vi "Service.vi"() -> ()   [LabVIEW 2019, in "Service.lvlib"]
uses:
  Service.lvlib
  mmw_command_lib/src_LabVIEW/mmW_commands/TypeDefs/commands.ctl
  TypeDef/AppStates.ctl
  mmw_instr_app_api/instr app state.ctl
  <vilib>/Field R&D Services/Logger/Type Definitions/Severity.ctl
  MsgQ/TypeDefs/CommandsQ.ctl
  MsgQ/TypeDefs/MsgQ_Commands.ctl
  mmw_command_lib/src_LabVIEW/mmW_commands/TypeDefs/response status.ctl
  <vilib>/Field R&D Services/Logger/Support/Create Level String.vi
  <vilib>/Field R&D Services/Logger/Support/Strip Whitespace.vi
  <vilib>/dlg_ctls.llb/Space Constant.vi
  <vilib>/Utility/error.llb/Trim Whitespace.vi
  <vilib>/Field R&D Services/Logger/Support/Manager.vi
  mmw_command_lib/src_LabVIEW/mmW_commands/commands/extract_messages/extract_configure_fs.vi
  mmw_command_lib/src_LabVIEW/mmW_commands/commands/extract_messages/extract_get_instrument_status.vi
  mmw_command_lib/src_LabVIEW/mmW_commands/commands/construct_messages/construct_get_instrument_status.vi
  <vilib>/Field R&D Services/Logger/Support/Control State.vi
  MsgQ/MsgQ.lvlib
  <vilib>/Field R&D Services/Logger/Field_RnD_Services_Logger_Toolkit.lvlib
  mmw_command_lib/src_LabVIEW/mmW_commands/mmW_commands.lvlib
  zmq_multipart_lib/src_LabVIEW/zmq_mulipart_lib/zmq_multipart_lib.lvclass
  mmw_instr_app_api/mmW_instr_app_API.lvlib
panel:
  in  "send":bool
  out "Array":T1[](array[typedef])
  in  "stop?":bool
  in  "Tab Control":enum32{"Server setup", "Debug", "Test Commands"}(tab)=enum."Debug"
  out "error out":errorcluster
  out "Main INI path":string="C:\\ProgramData\\Noffz\\mmW_Service\\mmw_Service.ini"
  out "Messages":i32(listbox)
  in  "Send Command":bool
  in  "commands":T2=enum."configure_rf"
  out "fc (Hz)":dbl
  out "parts":string[](array[string])
  out "state":T3
  out "watchdog timer":timestamp
  # "NI mmWave Service Application"
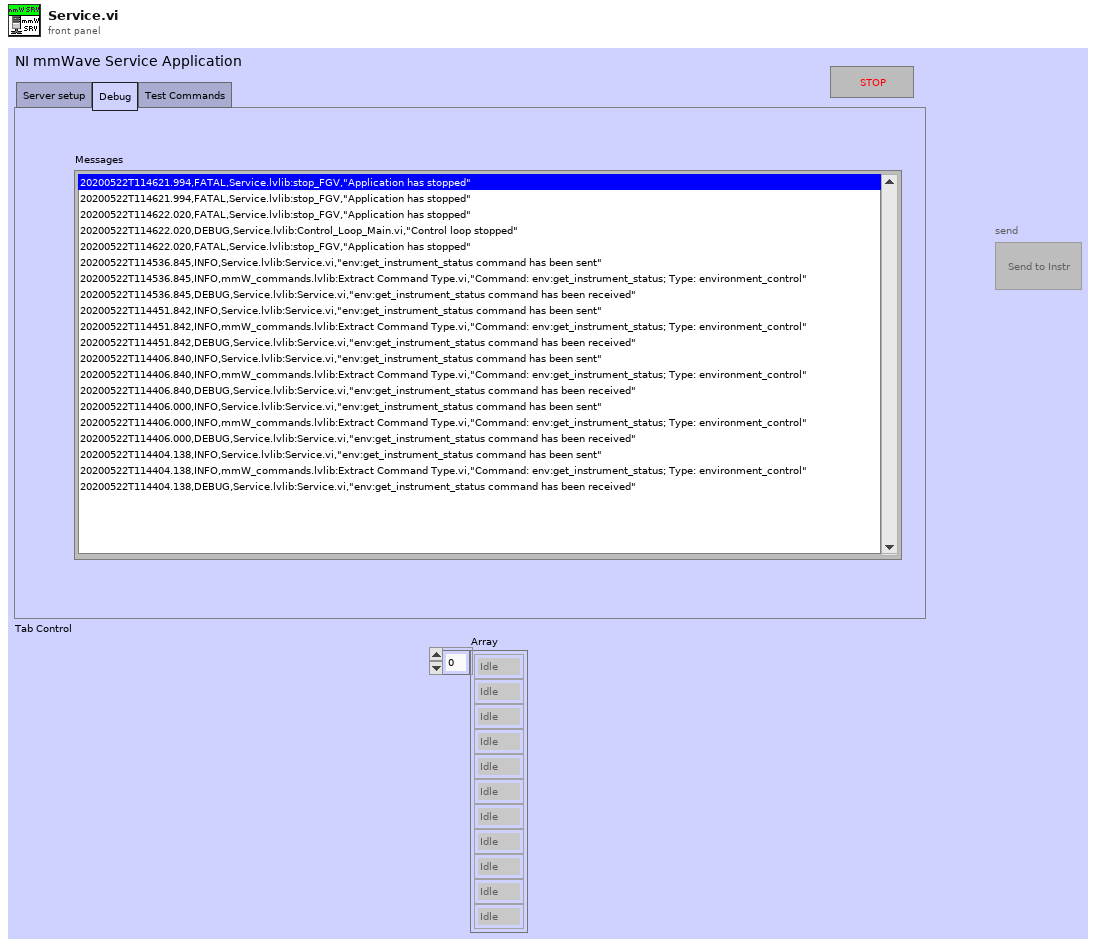
[diagram p1: front panel]
types:
  T1 = typedef "Service.lvlib/AppStates.ctl" = enum16{"Idle", "Init", "Proc_ZMQ_command", "Send_manual_command", "Shutdown", "Stop"}
  T2 = typedef "mmW_commands.lvlib/commands.ctl" = enum16{"configure_fs", "configure_rf", "configure_trigger", "equalization_enable", "equalization_start", "lo_sync_enable", "equalization_stop", "get_instrument_status", "get_versions", "initialize_hw", "pop_rx", "set_log_level", "Shutdown", "start", "start_instrument_app", "stop", "trans", "transceive", "trigger_burst", "trigger_sync_enable", "Write TX", "resp_generic", "resp_waveform", "send_trigger", "fetch", "transceive2"}
  T3 = typedef "mmW_instr_app_API.lvlib/instr app state.ctl" = enum16{"Off", "Initialization", "Configuration", "Running", "Calibration"}
  T4 = typedef "Field_RnD_Services_Logger_Toolkit.lvlib/Severity.ctl" = enum16{"Benign", "Warning", "Recoverable", "Fatal"}
  T5 = typedef "Service.lvlib/AppData.ctl" = cluster{"MsgQ":refnum<queue>, "Stop?":bool, "zmq sessions":cluster{"Control_endpoint":string, "Instr_endpoint":string}, "control-loop":cluster{"fromUI-Q":refnum<queue>, "toUI":refnum<user-event>, "Control_endpoint":string}, "UI-loop":cluster{"evnt_ref":refnum<event-registration>}, "logging":cluster{"level":dbl, "verbosity":dbl, "path":string, "Listener_ID":string}, "general_settings":cluster{"mmW_instr_ini_path":string, "mmW_instr_pid_path":string}}
  T6 = typedef "mmW_commands.lvlib/response status.ctl" = enum16{"OK", "Error", "Warning", "Unknown"}
  T7 = typedef "Service.lvlib/CommandsQ.ctl" = cluster{"cmd":T8, "data":variant, "notif":string}
  T8 = typedef "MsgQ.lvlib/MsgQ_Commands.ctl" = enum16{"message1", "message2", "message3", "generic", "transparent", "exception", "stop"}
  T9 = typedef "mmW_commands.lvlib/command_types.ctl" = enum16{"invalid_command", "instrument_control", "environment_control", "response"}
  T10 = typedef "Logger.lvlib/Statement.ctl" = cluster{"Time Stamp":timestamp, "Tag":T11, "Source":string, "Message":string}
  T11 = typedef "Logger.lvlib/Tag.ctl" = enum16{"Fatal", "Error", "Warn", "Info", "Debug", "Trace"}
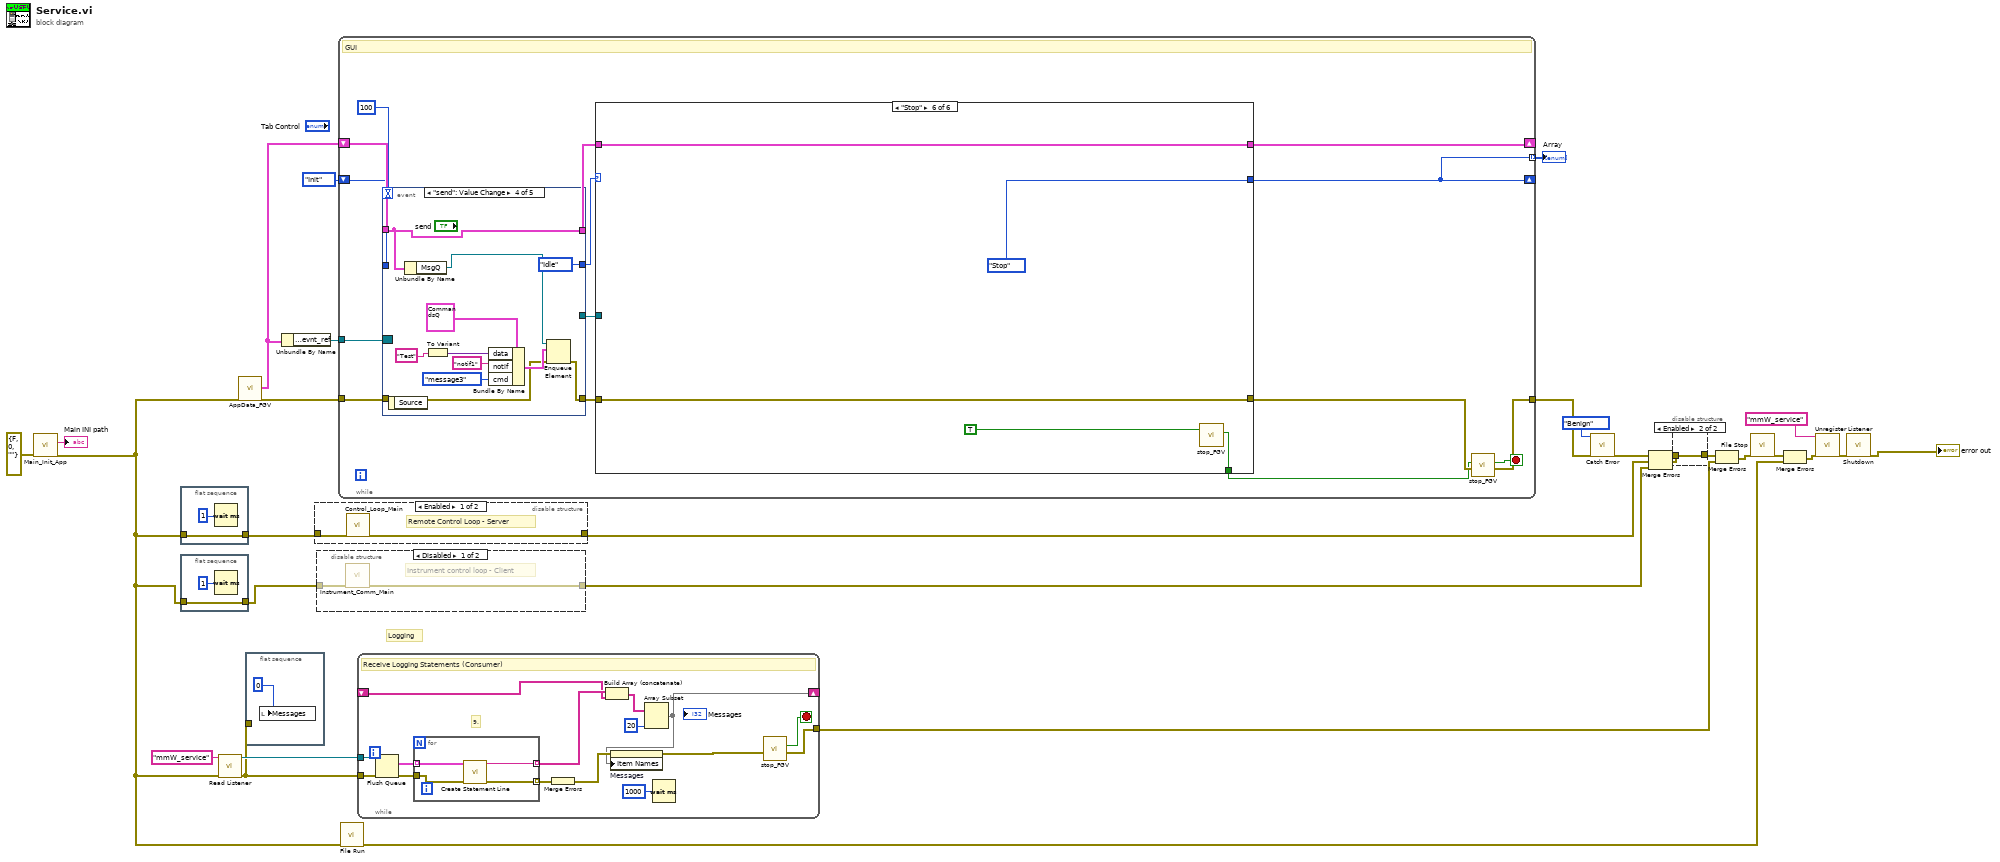
[diagram p0: block diagram]
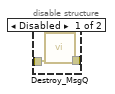
[diagram p3: hidden frame]
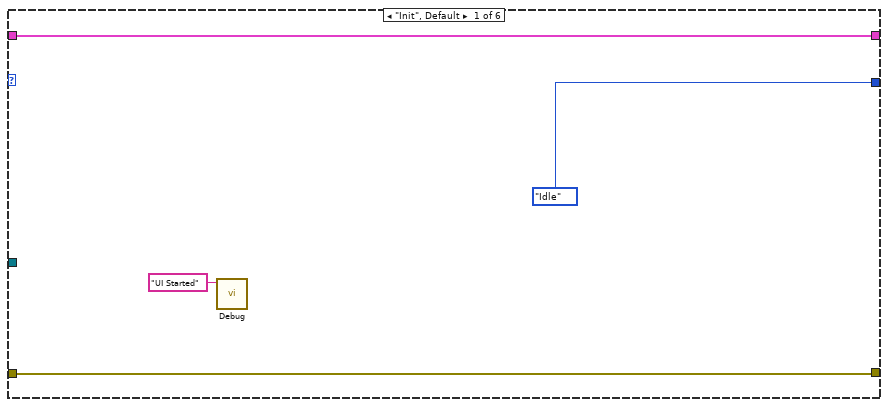
[diagram p5: hidden frame]
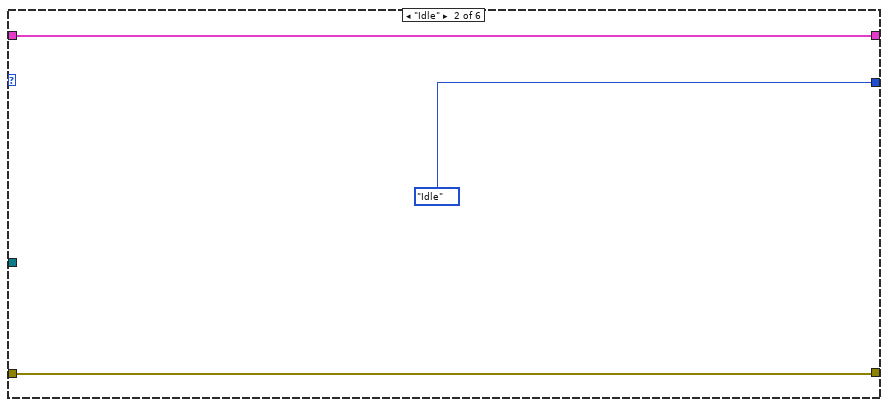
[diagram p6: hidden frame]
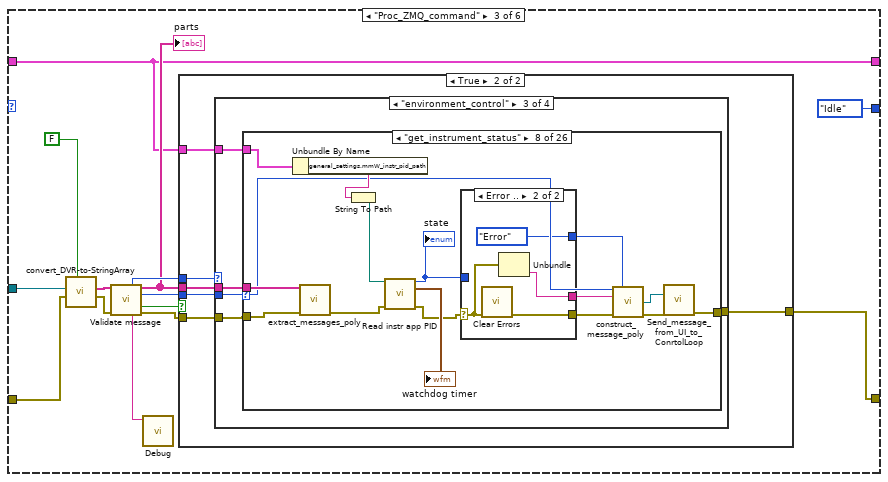
[diagram p7: hidden frame]
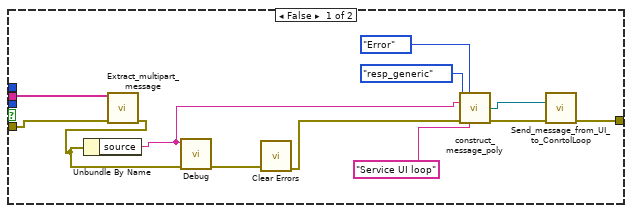
[diagram p8: hidden frame]
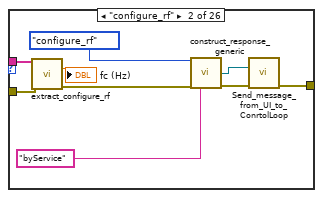
[diagram p12: hidden frame]
diagram:
  # "Logging"
  n1 = call "Main_Init_App.vi"("error in (no error)"=errorcluster {"status"=FALSE, "code"=0, "source"=""} ("Error In")) -> ("error out"=w3:errorcluster, "Main ini path"=→"Main INI path":string)  [unwired: 9 in]
  n2 = flat-sequence {
    tunnel: w3 -> [w30]
    tunnel: [w30] -> w4
    frame #0 {
      n3 = Wait (ms)(milliseconds to wait=u32 1) -> ()  [unwired: 1 out]
    }
  }
  n4 = flat-sequence {
    tunnel: w3 -> [w32]
    tunnel: [w32] -> w2
    frame #0 {
      n5 = Wait (ms)(milliseconds to wait=u32 1) -> ()  [unwired: 1 out]
    }
  }
  n6 = call <vilib>:"Read Listener.vi"("Error In"=w3, "Listener ID"="mmW_service") -> ("Error Out"=w9:errorcluster, "Listener"=w17:refnum<queue>)  [unwired: 8 in]
  n7 = call "AppData_FGV.vi"("error in (no error)"=w3) -> ("AppData out"=w8:T5, "error out"=w12:errorcluster)  [unwired: 17 in]
  n8 = flat-sequence {
    tunnel: w9 -> [_]
    frame #0 {
      n9 = local write "Messages"(0 ("Messages")) -> ()
    }
  }
  n10 = Unbundle By Name(w8) -> ("UI-loop.evnt_ref"=w7:refnum<event-registration>)
  n11 = disable-structure shown="Enabled" {
    disable-tunnel: [w35 w36] -> w20
    disable-tunnel: w4 -> [w34 w36]
    frame Enabled {
      # "Remote Control Loop - Server"
      n12 = call "Control_Loop_Main.vi"("error in (no error)"=w34) -> ("error out"=w35:errorcluster)  [unwired: 8 in, 2 out]
    }
    frame Disabled {
    }
  }
  n13 = disable-structure shown="Disabled" {
    disable-tunnel: [w38 w39] -> w19
    disable-tunnel: w2 -> [w37 w39]
    frame Disabled {
      # "Instrument control loop - Client"
      n14 = call "Instrument_Comm_Main.vi"("error in (no error)"=w37) -> ("error out"=w38:errorcluster)  [unwired: 10 in]
    }
    frame Enabled {
    }
  }
  n15 = while {
    tunnel: w12 -> [w45]
    tunnel: [w53] -> w22
    tunnel: w7 -> [w51]
    shift-right: [w40] -> _
    shift-left: AppStates."Init" ("States") -> [w41]
    shift-right: [w42] -> _
    shift-left: w8 -> [w44]
    tunnel: [w40] -> w5 mode=indexing
    stop <- w52 stop-if-true
    # "GUI"
    n16 = event shown="[3] \"send\": Value Change" {
      selector: w51 -> [_ _ _ _ _]
      dyn-events: _ -> [_ _ _ _ _]
      timeout: 100 -> [_ _ _ _ _]
      tunnel: w45 -> [w208 w209 w215 w220 w229]
      tunnel: [w208 w209 w215 w219 w229] -> w43
      tunnel: w44 -> [w206 w211 w212 w217 w228]
      tunnel: [_ _ w214 _ _] -> w49
      tunnel: [AppStates."Shutdown" ("States") AppStates."Send_manual_command" ("States") AppStates."Proc_ZMQ_command" ("States") AppStates."Idle" ("States") w227] -> w48
      tunnel: [w206 w211 w212 w217 w228] -> w46
      tunnel: w41 -> [_ _ _ _ w227]
      event "stop?": Value Change {
        n17 = event-data() -> ()  [unwired: 1 in, 1 out]
      }
      event "Send Command": Value Change {
        n18 = event-data() -> ()  [unwired: 1 in, 1 out]
      }
      event User Event {
        (unwired) refnum<data-value> refnum ("data value reference")
        n19 = event-data() -> ("data value reference"=w214:refnum<data-value>)  [unwired: 1 in, 4 out]
      }
      event "send": Value Change {
        n20 = event-data() -> ()  [unwired: 1 in, 1 out]
        n21 = Unbundle By Name(w217) -> ("MsgQ"=w216:refnum<queue>)
        n22 = To Variant(anything="Test" ("notif")) -> (Variant=w225:variant)
        n23 = Bundle By Name(cluster=T7 {"cmd"=enum."message1", "data"=variant, "notif"=""}, "data"=w225, "notif"="notif1", "cmd"=enum16{"message1", "message2", "message3"}."message3") -> (w224:T7)
        n24 = Enqueue Element(queue=w216, element=w224, error in (no error)=w220) -> (error out=w219:errorcluster)  [unwired: 1 in, 2 out]
      }
      event Timeout {
        n25 = event-data() -> ()  [unwired: 1 in, 1 out]
      }
    }
    n26 = case shown="\"Stop\"" w48 {
      tunnel: [w56 w60 w62 w191 w199 w203] -> w50
      tunnel: w49 -> [_ _ w74 _ _ _]
      tunnel: [AppStates."Idle" ("States") AppStates."Idle" ("States") AppStates."Idle" ("States") AppStates."Idle" ("States") AppStates."Stop" ("States") AppStates."Stop" ("States")] -> w40
      tunnel: [_ _ _ _ _ w204] -> w47
      tunnel: w46 -> [w55 w59 w63 w193 w198 w202]
      tunnel: w43 -> [w56 w60 w72 _ w199 w203]
      tunnel: [w55 w59 w63 w193 w198 w202] -> w42
      frame "Init", Default {
        n27 = call <vilib>:"Debug.vi"("Message"="UI Started") -> ()  [unwired: 10 in, 1 out]
      }
      frame "Idle" {
      }
      frame "Proc_ZMQ_command" {
        n28 = call "convert_DVR-to-StringArray.vi"("Delete DVR? (T)"=FALSE, "error in (no error)"=w72, "multipart message DVR in"=w74) -> ("error out"=w73:errorcluster, "parts"=w68:string[])  [unwired: 5 in]
        "parts" <- w68
        n29 = call "Validate message.vi"("multipart message in"=w68, "error in (no error)"=w73) -> ("Command Type"=w70:T9, "command out"=w69:T2, "Valid message?"=w71:bool, "Debug info"=w64:string, "error out"=w67:errorcluster)  [unwired: 8 in, 1 out]
        n30 = call <vilib>:"Debug.vi"("Message"=w64) -> ()  [unwired: 10 in, 1 out]
        n31 = case shown="True" w71 {
          tunnel: w70 -> [_ w92]
          tunnel: w69 -> [_ w91]
          tunnel: w68 -> [w85 w90]
          tunnel: w67 -> [w84 w89]
          tunnel: [w75 w87] -> w62
          tunnel: w63 -> [_ w88]
          frame False {
            n32 = call "Extract_multipart_message.vi"("multipart message in"=w85, "error in (no error)"=w84) -> ("error out"=w83:errorcluster)  [unwired: 6 in, 7 out]
            n33 = Unbundle By Name(w83) -> ("source"=w80:string)
            n34 = call <vilib>:"Debug.vi"("Error In"=w83, "Message"=w80) -> ("Error Out"=w86:errorcluster)  [unwired: 9 in]
            n35 = call <vilib>:"Clear Errors.vi"("error in (no error)"=w86) -> ("error out"=w79:errorcluster)  [unwired: 5 in, 1 out]
            n36 = call-poly "construct_message_poly.vi"("command in"=commands."resp_generic", "Status"=response_status."Error", "generic_info"=w80, "error in (no error) 2"=w79, "source"="Service UI loop") -> ("Multipart message DVR out"=w77:refnum<data-value>, "error out 2"=w76:errorcluster)  [unwired: 7 in, 2 out]
            n37 = call "Send_message_from_UI_to_ConrtolLoop.vi"("data DVR in"=w77, "error in (no error)"=w76) -> ("error out"=w75:errorcluster)  [unwired: 13 in]
          }
          frame True {
            n38 = case shown="\"environment_control\"" w92 {
              tunnel: w91 -> [_ w97 w136 _]
              tunnel: w90 -> [_ w96 w135 _]
              tunnel: w89 -> [w93 w95 w134 w188]
              tunnel: [w93 w94 w133 w188] -> w87
              tunnel: w88 -> [_ _ w132 _]
              frame "invalid_command", Default {
              }
              frame "instrument_control" {
                n39 = case shown="\"equalization_enable\"" w97 {
                  tunnel: w96 -> [_ w107 _ _ _ _ _ _ _ _ _ _ _ _ _ _ _ _ _ _ _ _ _ _ _ _]
                  tunnel: w95 -> [w98 w103 w108 w109 w110 w111 w112 w113 w114 w115 w116 w117 w118 w119 w120 w121 w122 w123 w124 w125 w126 w127 w128 w129 w130 w131]
                  tunnel: [w98 w99 w108 w109 w110 w111 w112 w113 w114 w115 w116 w117 w118 w119 w120 w121 w122 w123 w124 w125 w126 w127 w128 w129 w130 w131] -> w94
                  frame "configure_fs", Default {
                  }
                  frame "configure_rf" {
                    n40 = call "extract_configure_rf.vi"("multipart message in"=w107, "error in (no error)"=w103) -> ("fc (Hz)"=→"fc (Hz)":dbl, "error out"=w106:errorcluster)  [unwired: 8 in, 4 out]
                    n41 = call "construct_response_generic.vi"("command in"=commands."configure_rf", "error in (no error) 2"=w106, "source"="byService" ("generic_info")) -> ("Multipart message DVR out"=w100:refnum<data-value>, "error out 2"=w101:errorcluster)  [unwired: 9 in, 2 out]
                    n42 = call "Send_message_from_UI_to_ConrtolLoop.vi"("data DVR in"=w100, "error in (no error)"=w101) -> ("error out"=w99:errorcluster)  [unwired: 13 in]
                  }
                  frame "configure_trigger" {
                  }
                  frame "equalization_enable" {
                  }
                  frame "equalization_start" {
                  }
                  frame "lo_sync_enable" {
                  }
                  frame "equalization_stop" {
                  }
                  frame "get_instrument_status" {
                  }
                  frame "get_versions" {
                  }
                  frame "initialize_hw" {
                  }
                  frame "pop_rx" {
                  }
                  frame "set_log_level" {
                  }
                  frame "Shutdown" {
                  }
                  frame "start" {
                  }
                  frame "start_instrument_app" {
                  }
                  frame "stop" {
                  }
                  frame "trans" {
                  }
                  frame "transceive" {
                  }
                  frame "trigger_burst" {
                  }
                  frame "trigger_sync_enable" {
                  }
                  frame "Write TX" {
                  }
                  frame "resp_generic" {
                  }
                  frame "resp_waveform" {
                  }
                  frame "send_trigger" {
                  }
                  frame "fetch" {
                  }
                  frame "transceive2" {
                  }
                }
              }
              frame "environment_control" {
                n43 = case shown="\"get_instrument_status\"" w136 {
                  selector: w136 -> [_ _ _ _ _ _ _ w151 _ _ _ _ _ _ _ _ _ _ _ _ _ _ _ _ _ _]
                  tunnel: w135 -> [_ w139 _ _ _ _ _ w160 _ _ _ _ _ _ _ _ _ _ _ _ _ _ _ _ _ _]
                  tunnel: w134 -> [w137 w138 w140 w141 w142 w143 w144 w159 w170 w171 w172 w173 w174 w175 w176 w177 w178 w179 w180 w181 w182 w183 w184 w185 w186 w187]
                  tunnel: [w137 w138 w140 w141 w142 w143 w144 w152 w170 w171 w172 w173 w174 w175 w176 w177 w178 w179 w180 w181 w182 w183 w184 w185 w186 w187] -> w133
                  tunnel: w132 -> [_ _ _ _ _ _ _ w158 _ _ _ _ _ _ _ _ _ _ _ _ _ _ _ _ _ _]
                  frame "configure_fs", Default {
                    n44 = call-poly "extract_messages_poly.vi"() -> ()  [unwired: 11 in, 5 out]
                  }
                  frame "configure_rf" {
                    n45 = call-poly "extract_messages_poly.vi"("multipart message in"=w139) -> ()  [unwired: 9 in, 6 out]
                  }
                  frame "configure_trigger" {
                  }
                  frame "equalization_enable" {
                  }
                  frame "equalization_start" {
                  }
                  frame "lo_sync_enable" {
                  }
                  frame "equalization_stop" {
                  }
                  frame "get_instrument_status" {
                    n46 = Unbundle By Name(w158) -> ("general_settings.mmW_instr_pid_path"=w157:string)
                    n47 = call-poly "extract_messages_poly.vi"("multipart message in"=w160, "error in (no error)"=w159) -> ("error out"=w155:errorcluster)  [unwired: 11 in, 2 out]
                    n48 = String To Path(string=w157) -> (path=w156:path)
                    n49 = call "Read instr app PID.vi"("Path"=w156, "error in"=w155) -> ("state"=w150:T3, "watchdog timer"=→"watchdog timer":timestamp, "error out"=w147:errorcluster)  [unwired: 11 in]
                    "state" <- w150
                    n50 = case shown="Error .." w147 {
                      selector: w147 -> [w162 w167]
                      tunnel: w150 -> [w164 _]
                      tunnel: [w163 w166] -> w149
                      tunnel: [w162 w169] -> w146
                      tunnel: [response_status."OK" ("Status") response_status."Error" ("Status")] -> w145
                      frame No Error {
                        n51 = To Variant(anything=w164) -> (Variant=w165:variant)
                        n52 = call <userlib>:"Get Strings from Enum__ogtk.vi"("Enum"=w165) -> ("String Value"=w163:string)  [unwired: 7 in, 3 out]
                      }
                      frame Error {
                        n53 = call <vilib>:"Clear Errors.vi"("error in (no error)"=w167) -> ("error out"=w169:errorcluster)  [unwired: 5 in, 1 out]
                        n54 = Unbundle(w167) -> ("source"=w166:string)  [unwired: 2 out]
                      }
                    }
                    n55 = call-poly "construct_message_poly.vi"("command in"=w151, "Status"=w145, "generic_info"=w149, "error in (no error) 2"=w146) -> ("Multipart message DVR out"=w148:refnum<data-value>, "error out 2"=w153:errorcluster)  [unwired: 8 in, 2 out]
                    n56 = call "Send_message_from_UI_to_ConrtolLoop.vi"("data DVR in"=w148, "error in (no error)"=w153) -> ("error out"=w152:errorcluster)  [unwired: 13 in]
                  }
                  frame "get_versions" {
                  }
                  frame "initialize_hw" {
                  }
                  frame "pop_rx" {
                  }
                  frame "set_log_level" {
                  }
                  frame "Shutdown" {
                  }
                  frame "start" {
                  }
                  frame "start_instrument_app" {
                  }
                  frame "stop" {
                  }
                  frame "trans" {
                  }
                  frame "transceive" {
                  }
                  frame "trigger_burst" {
                  }
                  frame "trigger_sync_enable" {
                  }
                  frame "Write TX" {
                  }
                  frame "resp_generic" {
                  }
                  frame "resp_waveform" {
                  }
                  frame "send_trigger" {
                  }
                  frame "fetch" {
                  }
                  frame "transceive2" {
                  }
                }
              }
              frame "response" {
              }
            }
          }
        }
      }
      frame "Send_manual_command" {
        (unwired) u32 500 ("timeout (ms)")
        n57 = case shown="\"get_instrument_status\"" "commands" {
          tunnel: [_ _ _ _ _ _ _ w197 _ _ _ _ _ _ _ _ _ _ _ _ _ _ _ _ _ _] -> w189
          frame "configure_fs", Default {
          }
          frame "configure_rf" {
          }
          frame "configure_trigger" {
          }
          frame "equalization_enable" {
          }
          frame "equalization_start" {
          }
          frame "lo_sync_enable" {
          }
          frame "equalization_stop" {
          }
          frame "get_instrument_status" {
            n58 = call-poly "construct_message_poly.vi"("DVR/string output? (DVR=T)"=TRUE) -> ("data value reference"=w195:refnum<data-value>, "Debug info"=w197:string, "error out"=w194:errorcluster)  [unwired: 10 in, 2 out]
            n59 = call "Send_message_to_UI.vi"("Data Value Reference in"=w195, "error in (no error)"=w194) -> ()  [unwired: 13 in, 1 out]
          }
          frame "get_versions" {
          }
          frame "initialize_hw" {
          }
          frame "pop_rx" {
          }
          frame "set_log_level" {
          }
          frame "Shutdown" {
          }
          frame "start" {
          }
          frame "start_instrument_app" {
          }
          frame "stop" {
          }
          frame "trans" {
          }
          frame "transceive" {
          }
          frame "trigger_burst" {
          }
          frame "trigger_sync_enable" {
          }
          frame "Write TX" {
          }
          frame "resp_generic" {
          }
          frame "resp_waveform" {
          }
          frame "send_trigger" {
          }
          frame "fetch" {
          }
          frame "transceive2" {
          }
        }
        n60 = call <vilib>:"Info.vi"("Message"=w189) -> ("Error Out"=w191:errorcluster)  [unwired: 10 in]
      }
      frame "Shutdown" {
      }
      frame "Stop" {
        n61 = call "stop_FGV"("stop"=TRUE) -> ("stop?"=w204:bool)  [unwired: 7 in, 1 out]
      }
    }
    n62 = call "stop_FGV"("error in (no error)"=w50, "stop"=w47) -> ("error out"=w53:errorcluster, "stop?"=w52:bool)  [unwired: 6 in]
  }
  "Array" <- w5
  n63 = call <vilib>:"File Run.vi"("Error In"=w3) -> ("Error Out"=w28:errorcluster)  [unwired: 10 in]
  n64 = while {
    tunnel: w17 -> [w244]
    tunnel: w9 -> [w243]
    tunnel: [w230] -> w13
    shift-right: [w233] -> _
    shift-left: _ -> [w236]
    stop <- w231 stop-if-true
    # "9."
    # "Receive Logging Statements (Consumer)"
    n65 = Flush Queue(queue=w244, error in (no error)=w243) -> (remaining elements=w242:T10[], error out=w241:errorcluster)  [unwired: 1 out]
    n66 = for {
      tunnel: w242 -> [w248] mode=indexing
      tunnel: w241 -> [w247]
      tunnel: [w246] -> w237 mode=indexing
      tunnel: [w245] -> w240 mode=indexing
      n67 = call <vilib>:"Create Statement Line.vi"("Error In"=w247, "Statement"=w248) -> ("Error Out"=w245:errorcluster, "Line"=w246:string)  [unwired: 8 in]
    }
    n68 = Merge Errors(w240) -> (w239:errorcluster)
    n69 = Build Array (concatenate)(w237, w236) -> (w235:string[])
    n70 = Array Subset(array=w235, length=20) -> (w233:string[])  [unwired: 1 in]
    n71 = property on="Messages" class="LstBox (strict)"(error in=w239, "Item Names"=w233) -> (error out=w232:errorcluster)  [unwired: 1 in, 1 out]
    n72 = Wait (ms)(milliseconds to wait=u32 1000) -> ()  [unwired: 1 out]
    n73 = call "stop_FGV"("error in (no error)"=w232) -> ("error out"=w230:errorcluster, "stop?"=w231:bool)  [unwired: 7 in]
  }
  n74 = call <vilib>:"Catch Error.vi"("Error In"=w22, "Severity"=Severity."Benign") -> ("Error Out"=w21:errorcluster)  [unwired: 9 in]
  n75 = Merge Errors(w21, w20, w19) -> (w10:errorcluster)
  n76 = disable-structure shown="Enabled" {
    disable-tunnel: [w250 w251] -> w15
    disable-tunnel: w10 -> [w249 w251]
    frame Disabled {
      n77 = call "Destroy_MsgQ.vi"("error in (no error)"=w249) -> ("error out"=w250:errorcluster)  [unwired: 10 in]
    }
    frame Enabled {
    }
  }
  n78 = Merge Errors(w15, w13) -> (w14:errorcluster)
  n79 = call <vilib>:"File Stop.vi"("Error In"=w14) -> ("Error Out"=w24:errorcluster)  [unwired: 10 in]
  n80 = Merge Errors(w24, w28) -> (w27:errorcluster)
  n81 = call <vilib>:"Unregister Listener.vi"("Error In"=w27, "Listener ID"="mmW_service") -> ("Error Out"=w26:errorcluster)  [unwired: 9 in]
  n82 = call <vilib>:"Shutdown.vi"("Error In"=w26) -> ("Error Out"=→"error out":errorcluster)  [unwired: 10 in]
